vi "SimpleBox.vi"(0 "Box":cluster{"Length":sgl, "Width":sgl, "Height":sgl}={"Length"=0.4, "Width"=0.2, "Height"=0.1}, 1 "Name":string, 2 "origin":T2, 3 "mass":dbl=1.0, 4 "link color":u32(colorbox)=16712704) -> (5 "Link":T1)   [LabVIEW 2010]
uses:
  LINK.ctl
  Position.ctl
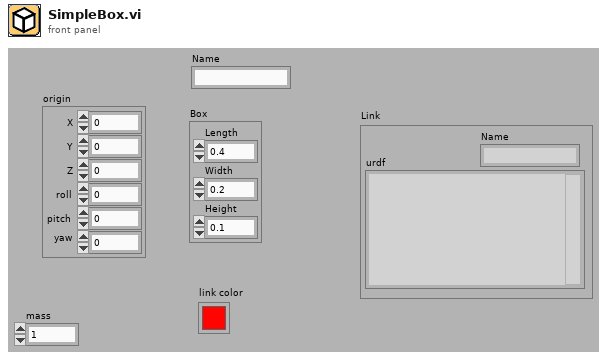
[diagram p1: front panel]
types:
  T1 = typedef "LINK.ctl" = cluster{"Name":string, "urdf":string}
  T2 = typedef "Position.ctl" = cluster{"X":sgl, "Y":sgl, "Z":sgl, "roll":sgl, "pitch":sgl, "yaw":sgl}
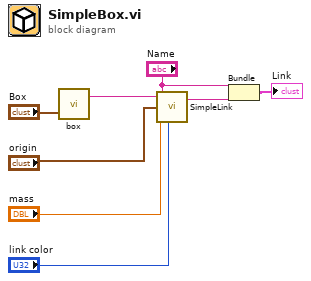
[diagram p0: block diagram]
diagram:
  n1 = call "box.vi"("Box"="Box") -> ("urdf out"=w5:string)  [unwired: 3 in]
  n2 = call "SimpleLink.vi"("Geometry"=w5, "Name"="Name", "origin"="origin", "mass"="mass", "link color"="link color") -> ("link out"=w3:string)  [unwired: 1 in]
  n3 = Bundle("Name"="Name", "link out"=w3) -> (→"Link":cluster{"Name":string, "link out":string})  [unwired: 1 in]
